vi "Read Animation Data.vi"(8 "error in (no error)":errorcluster, 11 "Animation Path":path) -> (0 "error out":errorcluster, 1 "Animation Set Name":string, 2 "Total Number of Frames":i32, 3 "Animation Reel":picture[](array[picture]))   [LabVIEW 2014]
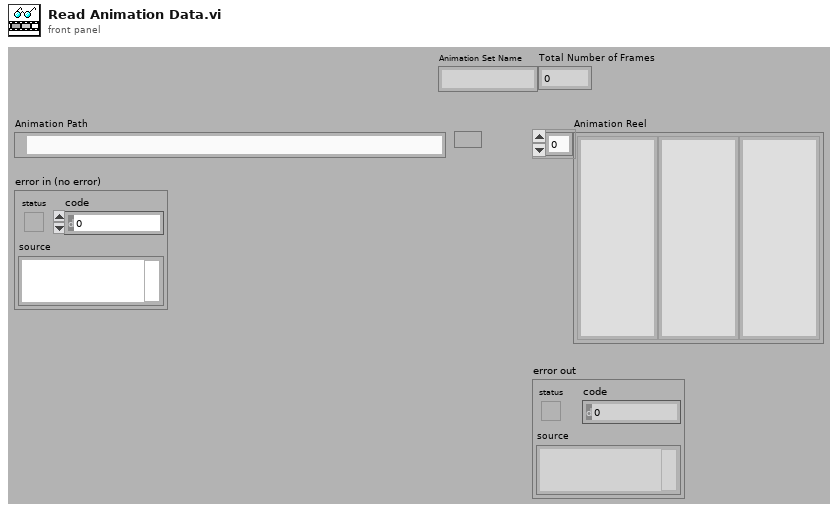
[diagram p1: front panel]
types:
  T1 = typedef "imagedata.ctl" = cluster{"image type":i32, "image depth":i32, "image":u8[], "mask":u8[], "colors":u32[], "Rectangle":cluster{"left":i16, "top":i16, "right":i16, "bottom":i16}}
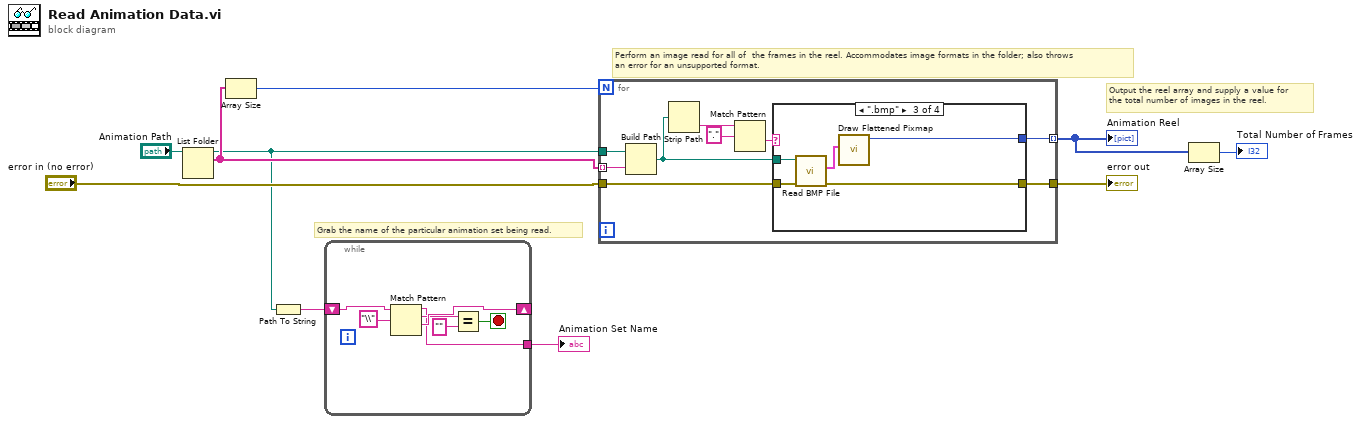
[diagram p0: block diagram]
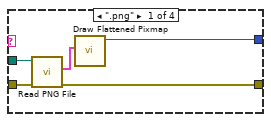
[diagram p2: hidden frame]
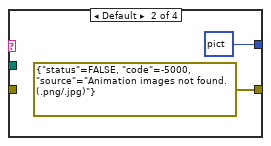
[diagram p3: hidden frame]
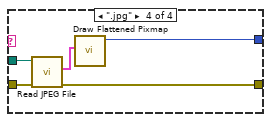
[diagram p4: hidden frame]
diagram:
  # "Output the reel array and supply a value for\nthe total number of images in the reel."
  # "Perform an image read for all of  the frames in the reel. Accommodates image formats in the folder; also throws\nan error for an unsupported format."
  # "Grab the name of the particular animation set being read."
  n1 = List Folder(path="Animation Path") -> (path out=w5:path, filenames=w6:string[])  [unwired: 3 in, 2 out]
  n2 = Array Size(array=w6) -> (size(s)=w8:i32)
  n3 = Path To String(path=w5) -> (string=w4:string)
  n4 = while {
    shift-right: [w15] -> _
    shift-left: w4 -> [w17]
    tunnel: [w11] -> w3
    stop <- w14 stop-if-true
    n5 = Match Pattern(string=w17, regular expression="\\") -> (before substring=w11:string, match substring=w13:string, after substring=w15:string)  [unwired: 1 in, 1 out]
    n6 = Equal?(x=w13, y="") -> (x = y?=w14:bool)
  }
  "Animation Set Name" <- w3
  n7 = for {
    N: w8 -> [_]
    tunnel: w6 -> [w26] mode=indexing
    tunnel: w5 -> [w25]
    tunnel: "error in (no error)" -> [w24]
    tunnel: [w23] -> w10
    tunnel: [w22] -> w2 mode=indexing
    n8 = Build Path(base path=w25, name or relative path=w26) -> (appended path=w21:path)
    n9 = Strip Path(path=w21) -> (name=w20:string)  [unwired: 1 out]
    n10 = Match Pattern(string=w20, regular expression=".") -> (after substring=w18:string)  [unwired: 1 in, 3 out]
    n11 = case shown="\".bmp\"" w18 {
      tunnel: [w30 errorcluster {"status"=FALSE, "code"=-5000, "source"="Animation images not found. (.png/.jpg)"} ("error in (no error)") w37 w42] -> w23
      tunnel: w24 -> [w31 _ w38 w43]
      tunnel: [w27 picture data[5B] ("new picture") w34 w39] -> w22
      tunnel: w21 -> [w29 _ w36 w41]
      frame ".png" {
        n12 = call <vilib>:"Read PNG File.vi"("error in (no error)"=w31, "path to PNG file"=w29) -> ("error out"=w30:errorcluster, "image data"=w28:T1)  [unwired: 7 in, 1 out]
        n13 = call <vilib>:"Draw Flattened Pixmap.vi"("image data"=w28) -> ("new picture"=w27:picture)  [unwired: 8 in]
      }
      frame Default {
      }
      frame ".bmp" {
        n14 = call <vilib>:"Read BMP File.vi"("error in (no error)"=w38, "path to BMP file"=w36) -> ("error out"=w37:errorcluster, "image data"=w35:T1)  [unwired: 7 in, 1 out]
        n15 = call <vilib>:"Draw Flattened Pixmap.vi"("image data"=w35) -> ("new picture"=w34:picture)  [unwired: 8 in]
      }
      frame ".jpg" {
        n16 = call <vilib>:"Read JPEG File.vi"("error in (no error)"=w43, "path to JPEG file"=w41) -> ("error out"=w42:errorcluster, "image data"=w40:T1)  [unwired: 7 in, 1 out]
        n17 = call <vilib>:"Draw Flattened Pixmap.vi"("image data"=w40) -> ("new picture"=w39:picture)  [unwired: 8 in]
      }
    }
  }
  "error out" <- w10
  "Animation Reel" <- w2
  n18 = Array Size(array=w2) -> (size(s)=→"Total Number of Frames":i32)
